vi "PXI-Zero 16-bit Outputs.vi"(8 "error in (no error)":errorcluster) -> (0 "error out":errorcluster)   [LabVIEW 2020]
uses:
  <vilib>/DAQmx/write.llb/DAQmx Write (Analog 2D DBL NChan NSamp).vi
  <vilib>/DAQmx/create/channels.llb/DAQmx Create Channel (AO-Voltage-Basic).vi
  <vilib>/DAQmx/configure/timing.llb/DAQmx Timing (Sample Clock).vi
  <vilib>/DAQmx/miscellaneous.llb/DAQmx Fill In Error Info.vi
  <resource>/objmgr/daqmx.rc
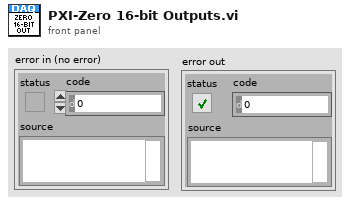
[diagram p1: front panel]
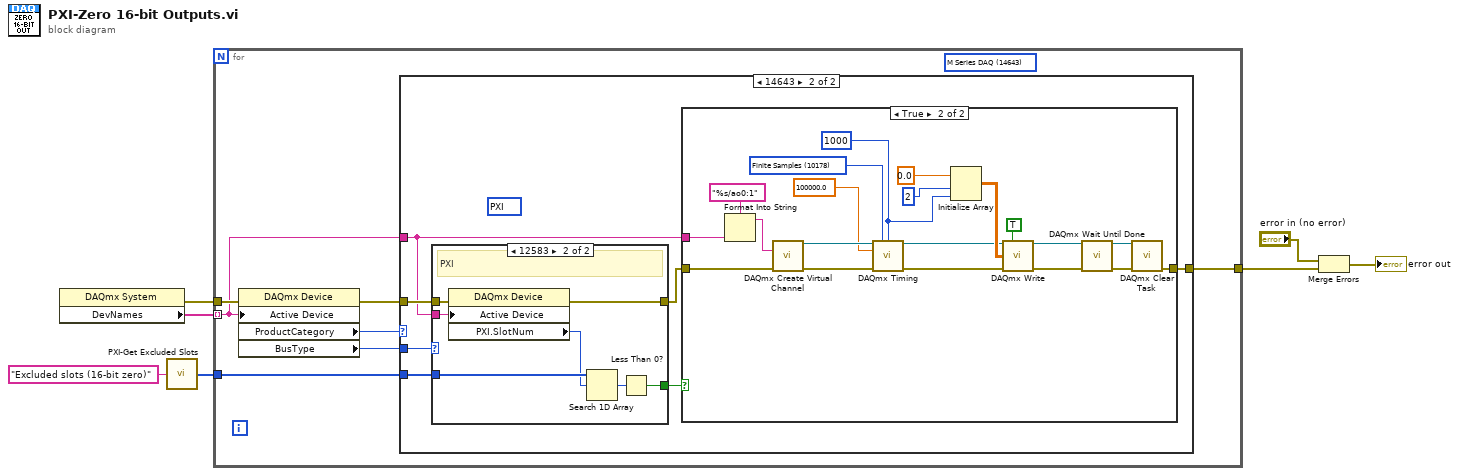
[diagram p0: block diagram]
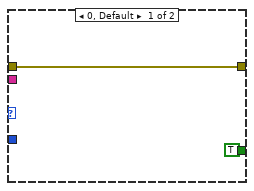
[diagram p3: hidden frame]
diagram:
  n1 = property class="DAQmx System"() -> (error out=w3:errorcluster, "DevNames"=w4:tag[])  [unwired: 2 in, 1 out]
  n2 = call "PXI-Get Excluded Slots.vi"("key"="Excluded slots (16-bit zero)") -> ("excluded slots"=w2:i32[])  [unwired: 13 in, 1 out]
  n3 = for {
    tunnel: w4 -> [w11] mode=indexing
    tunnel: w3 -> [w14]
    tunnel: [w12] -> w7
    tunnel: w2 -> [w8]
    (unwired) 14643 items=["M Series DAQ"=14643, "X Series DAQ"=15858, "E Series DAQ"=14642, "S Series DAQ"=14644, "B Series DAQ"=14662, "SC Series DAQ"=14645, "USB DAQ"=14646, "AO Series"=14647, "Digital I/O"=14648, "TIO Series"=14661, "Dynamic Signal Acquisition"=14649, "Switches"=14650, "CompactDAQ Chassis"=14658, "C Series Module"=14659, "SCXI Module"=14660, "SCC Connector Block"=14704, "SCC Module"=14705, "NI ELVIS"=14755, "Network DAQ"=14829, "SC Express"=15886, "Unknown"=12588] ("ProductCategory")
    n4 = property class="DAQmx Device"(error in=w14, "Active Device"=w11) -> (error out=w13:errorcluster, "ProductCategory"=w10:i32, "BusType"=w9:i32)  [unwired: 1 in, 1 out]
    n5 = case shown="14643" w10 {
      tunnel: w13 -> [_ w19]
      tunnel: [_ w21] -> w12
      tunnel: w11 -> [_ w18]
      tunnel: w9 -> [_ w20]
      tunnel: w8 -> [_ w16]
      frame 0, Default {
      }
      frame 14643 {
        (unwired) 12583 items=["PCI"=12582, "PCIe"=13612, "PXI"=12583, "PXIe"=14706, "SCXI"=12584, "SCC"=14707, "PCCard"=12585, "USB"=12586, "CompactDAQ"=14637, "TCP/IP"=14828, "Unknown"=12588, "SwitchBlock"=15870] ("BusType")
        n6 = case shown="12583" w20 {
          tunnel: w19 -> [w22 w30]
          tunnel: w18 -> [_ w29]
          tunnel: [w22 w28] -> w17
          tunnel: w16 -> [_ w27]
          tunnel: [TRUE w24] -> w15
          frame 0, Default {
          }
          frame 12583 {
            # "PXI"
            n7 = property class="DAQmx Device"(error in=w30, "Active Device"=w29) -> (error out=w28:errorcluster, "PXI.SlotNum"=w26:u32)  [unwired: 1 in, 1 out]
            n8 = Search 1D Array(1D array=w27, element=w26) -> (index of element=w25:i32)  [unwired: 1 in]
            n9 = Less Than 0?(x=w25) -> (x < 0?=w24:bool)
          }
        }
        n10 = case shown="True" w15 {
          tunnel: w17 -> [w31 w51]
          tunnel: [w31 w47] -> w21
          tunnel: w18 -> [_ w32]
          frame False {
          }
          frame True {
            w35 = 1000 ("samples per channel")
            w44 = 10178 items=["Finite Samples"=10178, "Continuous Samples"=10123, "Hardware Timed Single Point"=12522] ("sample mode")
            n11 = Format Into String(format string="%s/ao0:1" ("physical channels"), w32) -> (resulting string=w34:string)  [unwired: 2 in, 1 out]
            n12 = call-poly <vilib>:"DAQmx Create Virtual Channel.vi"("physical channels"=w34, "error in"=w51) -> ("task out"=w46:refnum<k21>, "error out"=w45:errorcluster)  [unwired: 12 in]
            n13 = call-poly <vilib>:"DAQmx Timing.vi"("task/channels in"=w46, "sample mode"=w44, "samples per channel"=w35, "rate"=100000.0, "error in"=w45) -> ("task out"=w38:refnum<k21>, "error out"=w37:errorcluster)  [unwired: 9 in]
            n14 = Initialize Array(0.0 ("element"), 2 ("dimension size"), w35) -> (w40:dbl[][])
            n15 = call-poly <vilib>:"DAQmx Write.vi"("task/channels in"=w38, "auto start"=TRUE, "data"=w40, "error in"=w37) -> ("task out"=w42:refnum<k21>, "error out"=w41:errorcluster)  [unwired: 9 in, 1 out]
            n16 = call <vilib>:"DAQmx Wait Until Done.vi"("task/channels in"=w42, "error in"=w41) -> ("task out"=w49:refnum<k21>, "error out"=w48:errorcluster)  [unwired: 12 in]
            n17 = call <vilib>:"DAQmx Clear Task.vi"("task in"=w49, "error in"=w48) -> ("error out"=w47:errorcluster)  [unwired: 13 in]
          }
        }
      }
    }
  }
  n18 = Merge Errors("error in (no error)", w7) -> (→"error out":errorcluster)
